vi "PRL SIGNAL Create Waveform Array.vi"(7 "Signal Names":string[](array[string]), 10 "Analog Signals":sgl[][](array[numeric]), 11 "Timestamp":timestamp[](array[timestamp])) -> (3 "Waveform Array":waveform(sgl)[](array[waveform]))   [LabVIEW 2013, in "PMU Recorder Light.lvlib"]
uses:
  PMU Recorder Light.lvlib
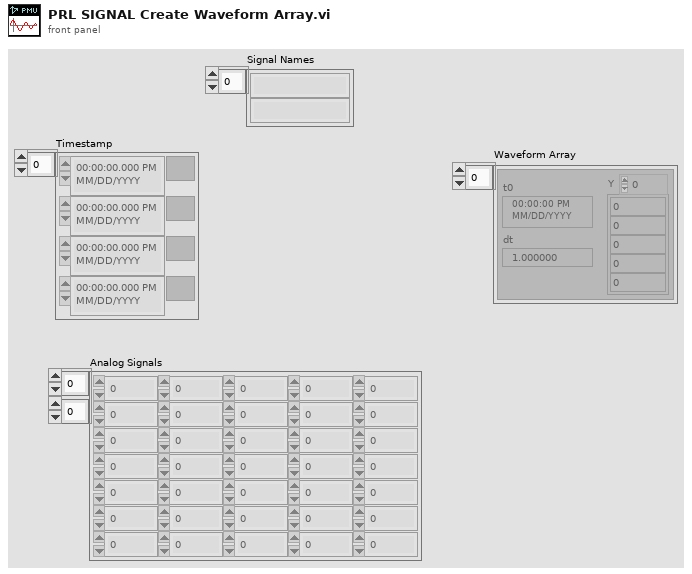
[diagram p1: front panel]
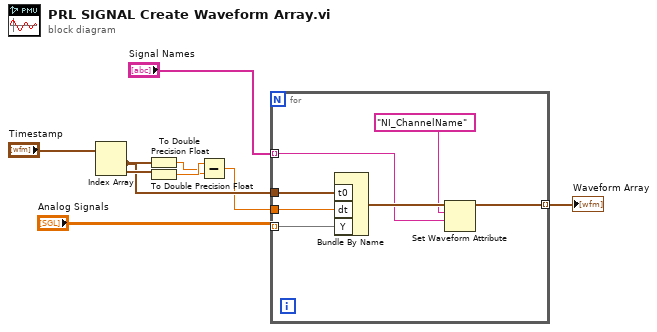
[diagram p0: block diagram]
diagram:
  n1 = Index Array(array="Timestamp") -> (element #1=w5:timestamp, element #2=w8:timestamp)  [unwired: 2 in]
  n2 = To Double Precision Float(number=w5) -> (double precision float=w6:dbl)
  n3 = To Double Precision Float(number=w8) -> (double precision float=w7:dbl)
  n4 = Subtract(x=w7, y=w6) -> (x-y=w4:dbl)
  n5 = for {
    tunnel: w5 -> [w16]
    tunnel: w4 -> [w15]
    tunnel: "Analog Signals" -> [w14] mode=indexing
    tunnel: "Signal Names" -> [w11] mode=indexing
    tunnel: [w10] -> w1 mode=indexing
    n6 = Bundle By Name("t0"=w16, "dt"=w15, "Y"=w14) -> (w13:waveform(sgl))  [unwired: 1 in]
    n7 = Set Waveform Attribute(5:w11, 6:"NI_ChannelName" ("name"), 7:w13) -> (3:w10:waveform(sgl))  [unwired: 1 in, 2 out]
  }
  "Waveform Array" <- w1
